vi "Entry.vi"(8 "error in (no error)":errorcluster, 11 "New State":refnum<class "COOKING.lvclass">) -> (0 "error out":errorcluster, 3 "State out":refnum<class "COOKING.lvclass">)   [LabVIEW 2021, in "Chef States.lvlib" / "COOKING.lvclass"]
doc: "This is an abstract method. Override this method to define the behavior when you enter the state."
uses:
  COOKING.lvclass
  Chef State/Chef State.lvclass
  <vilib>/ActorFramework/Actor/Actor.lvclass
  Root Actor Logic/Root Actor Logic Messages/Update State String Msg/Update State String Msg.lvclass
  Kitchen Actor/Kitchen Actor.lvclass
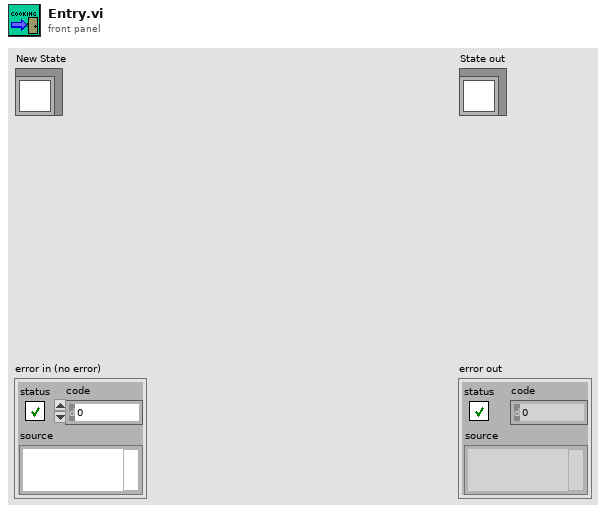
[diagram p1: front panel]
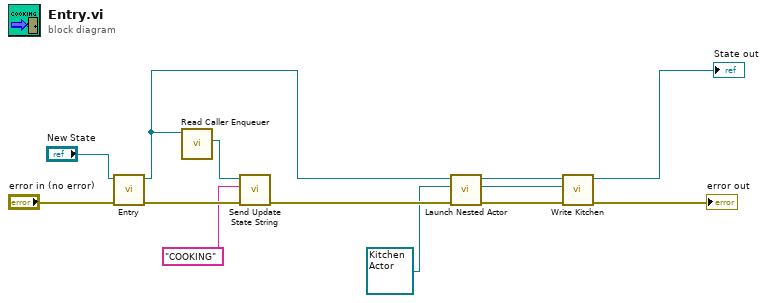
[diagram p0: block diagram]
diagram:
  n1 = call-parent "Entry.vi"("error in (no error)"="error in (no error)", "New State"="New State") -> ("error out"=w13:errorcluster, "State out"=w7:refnum<class "COOKING.lvclass">)  [unwired: 8 in]
  n2 = call <vilib>:"Read Caller Enqueuer.vi"("Actor"=w7) -> ("Caller Enqueuer"=w9:refnum<class "Message Enqueuer.lvclass">)  [unwired: 10 in]
  n3 = call "Send Update State String.vi"("error in (no error)"=w13, "State"="COOKING", "Message Enqueuer"=w9) -> ("error out"=w10:errorcluster)  [unwired: 7 in, 1 out]
  n4 = call <vilib>:"Launch Nested Actor.vi"("error in (no error)"=w10, "Nested Actor"=refnum<class "Kitchen Actor.lvclass"> refnum ("Kitchen Actor.lvlib:Kitchen Actor.lvclass"), "Caller Actor in"=w7) -> ("error out"=w4:errorcluster, "Nested Actor's Enqueuer"=w2:refnum<class "Message Enqueuer.lvclass">, "Caller Actor out"=w6:refnum<class "COOKING.lvclass">)  [unwired: 6 in]
  n5 = call-dynamic "Write Kitchen.vi"("error in (no error)"=w4, "Kitcher Message Enqueuer"=w2, "COOKING in"=w6) -> ("error out"=→"error out":errorcluster, "COOKING out"=→"State out":refnum<class "COOKING.lvclass">)  [unwired: 7 in]
